vi "parse_vector_search_response.vi"(0 "headers":string, 5 "body":string, 7 "collection name":string, 11 "error in (no error)":errorcluster) -> (4 "Data":cluster{"text":string}[](array[cluster]), 15 "error out":errorcluster)   [LabVIEW 2020, in "vector_weviate.lvclass"]
doc: "This VI parses the response of the Add Vector request"
uses:
  vector_weviate.lvclass
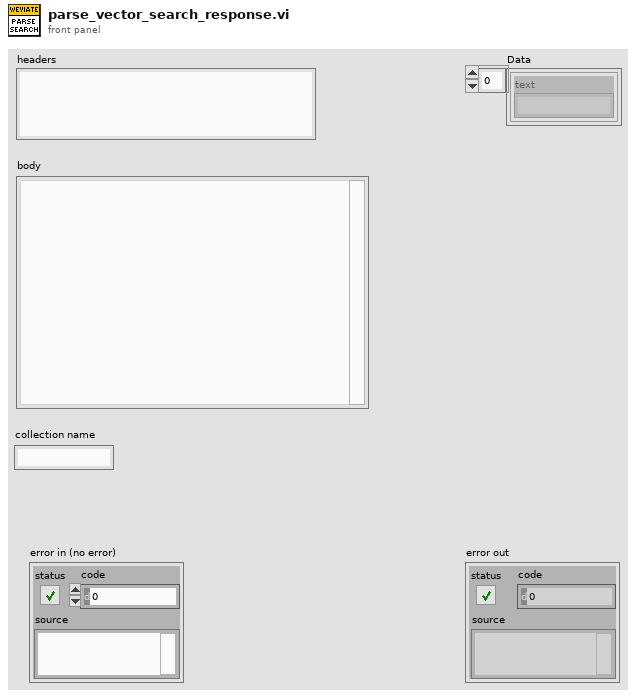
[diagram p1: front panel]
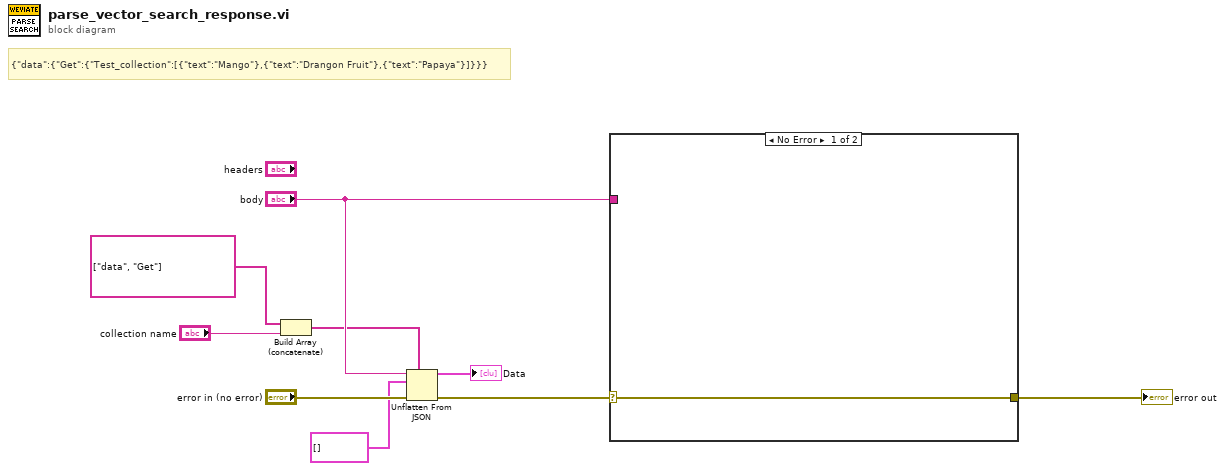
[diagram p0: block diagram]
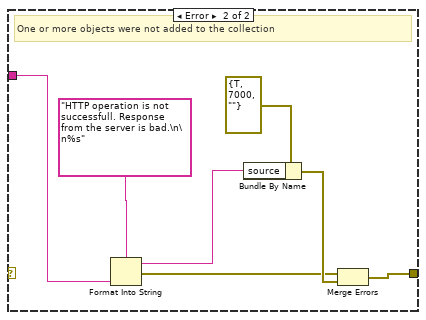
[diagram p2: hidden frame]
diagram:
  # "{\"data\":{\"Get\":{\"Test_collection\":[{\"text\":\"Mango\"},{\"text\":\"Drangon Fruit\"},{\"text\":\"Papaya\"}]}}}"
  n1 = Build Array (concatenate)(string[] ["data", "Get"] ("path"), "collection name") -> (w2:string[])
  n2 = Unflatten From JSON(path=w2, JSON string="body", type and defaults=cluster{"text":string}[] [], error in (no error)="error in (no error)") -> (value=→"Data":cluster{"text":string}[], error out=w8:errorcluster)  [unwired: 3 in]
  n3 = case shown="No Error" w8 {
    selector: w8 -> [w10 _]
    tunnel: [w10 w15] -> w7
    tunnel: "body" -> [_ w12]
    frame No Error {
    }
    frame Error {
      # "One or more objects were not added to the collection"
      n4 = Format Into String(format string="HTTP operation is not successfull. Response from the server is bad.\n\n%s", w12) -> (resulting string=w11:string, error out=w14:errorcluster)  [unwired: 2 in]
      n5 = Bundle By Name(cluster=errorcluster {"status"=TRUE, "code"=7000, "source"=""} ("error constant"), "source"=w11) -> (w16:errorcluster)
      n6 = Merge Errors(w14, w16) -> (w15:errorcluster)
    }
  }
  "error out" <- w7
